vi "rql_Update LCD.vi"(4 "Show in Debugger?":bool=TRUE, 6 "Message Priority":T1=enum."Normal", 8 "error in":errorcluster, 10 "Data in":T2, 11 "Front Panel Emulator in":refnum<class "Front Panel Emulator.lvclass">) -> (0 "error out":errorcluster, 3 "dup Front Panel Emulator out":refnum<class "Front Panel Emulator.lvclass">)   [LabVIEW 2017, in "Front Panel Emulator.lvclass"]
doc: "This VI sends a <b>Local API Request</b> message to an MHL case of the Worker that owns this VI.\n---\nUpdates the LCD display on the FP with the latest data."
uses:
  Front Panel Emulator.lvclass
  C:/Program Files (x86)/National Instruments/LabVIEW 2017/vi.lib/addons/_Workers/Library/Classes/Worker/Worker.lvclass
  rql_Update LCD.ctl
  <vilib>/addons/_Workers/Library/Classes/Message/Priority.ctl
  <vilib>/addons/_Workers/Library/Case Label.ctl
  <vilib>/addons/_Workers/Library/Classes/Message Queue/Message Queue.lvclass
  <vilib>/addons/_Workers/Library/Workers.lvlib
  <vilib>/addons/_Workers/Library/Classes/Message/Message.lvclass
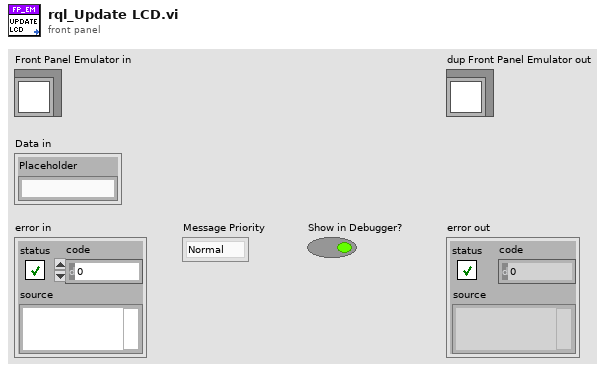
[diagram p1: front panel]
types:
  T1 = typedef "Workers.lvlib/Message.lvclass/Priority.ctl" = enum16{"Low", "Normal", "High"}
  T2 = typedef "Front Panel Emulator.lvclass/rql_Update LCD.ctl" = cluster{"Placeholder":string}
  T3 = typedef "Workers.lvlib/Case Label.ctl" = string
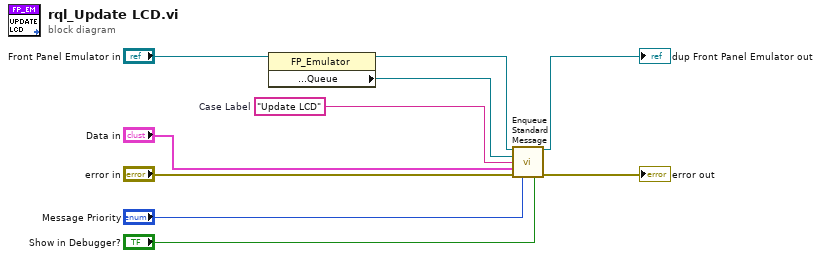
[diagram p0: block diagram]
diagram:
  w1 = T3 "Update LCD"  # Case Label
  n1 = property class="FP_Emulator"(reference="Front Panel Emulator in") -> (reference out=w3:refnum<class "Front Panel Emulator.lvclass">, "Accessors:Read:Public API:Queue"=w2:refnum<class "Message Queue.lvclass">)  [unwired: 1 in, 1 out]
  n2 = call-dynamic "Enqueue Standard Message.vi"("Worker"=w3, "Message Queue"=w2, "Case Label"=w1, "Data"="Data in", "error in (no error)"="error in", "Priority (Normal)"="Message Priority", "Send Message to Debugger? (T)"="Show in Debugger?") -> ("dup Worker out"=→"dup Front Panel Emulator out":refnum<class "Front Panel Emulator.lvclass">, "error out"=→"error out":errorcluster)  [unwired: 7 in]
